vi "ReportPart.vi"(6 "试验项目":T2(ring), 8 "error in":errorcluster, 9 "索引IN":i32, 10 "合格":T1, 11 "report in":refnum<class "NI_report.lvclass">) -> (0 "error out 2":errorcluster caption="error out", 2 "索引OUT":i32, 3 "report out":refnum<class "NI_report.lvclass">)   [LabVIEW 2020]
uses:
  <vilib>/Utility/NIReport.llb/NI_report.lvclass
  OK.ctl
  <vilib>/Utility/NIReport.llb/image depth.ctl
  <vilib>/addons/_office/_exclsub.llb/font.ctl
  Global_Variable/Global.vi
  Global_Variable/A180648.vi
  <vilib>/Utility/NIReport.llb/Append Report Text (str wrap).vi
  <vilib>/addons/_office/word.llb/Word Easy Table (str).vi
  <vilib>/Utility/NIReport.llb/NI_ReportGenerationCore.lvlib
  <vilib>/addons/_office/NI_ReportGenerationToolkit.lvlib
  <vilib>/Utility/NIReport.llb/Word/NI_Word.lvclass
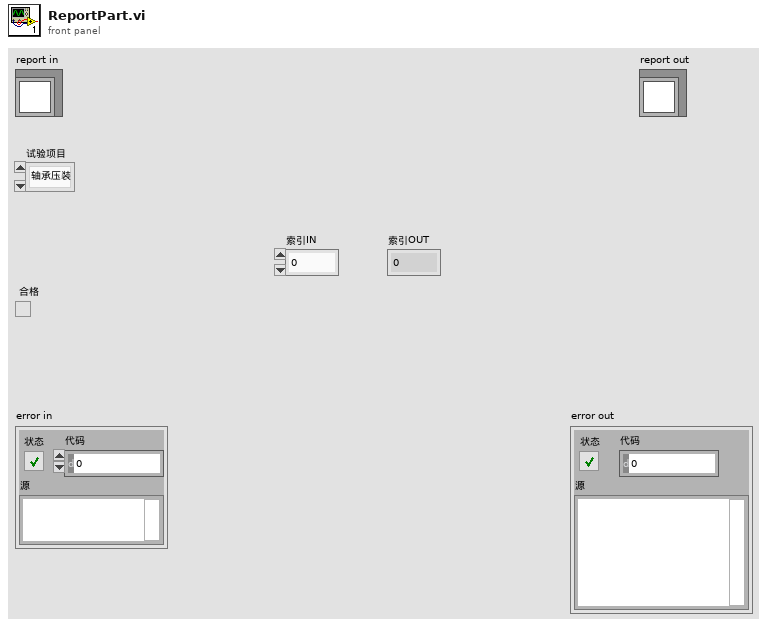
[diagram p1: front panel]
types:
  T1 = typedef "OK.ctl" = bool
  T2 = enum32{"轴承压装", "侧铆", "端铆", "电流特性", "传感器特性", "振动NVH", "磨合"}
  T3 = cluster{"Charset (-1)":i16, "Weight (-1)":i16, "Name":string, "Size":string}
  T4 = typedef "NI_ReportGenerationToolkit.lvlib/font.ctl" = cluster{"font name":string, "font size":dbl, "bold":u16, "italic":u16, "underline":u16, "strike through":u16, "font color":u32}
  T5 = cluster{"Italic":enum16{"Italic Unchanged", "Italic On", "Italic Off"}, "Strike Through":enum16{"Strike Through Unchanged", "Strike Through On", "Strike Through Off"}, "Underline":enum16{"Underline Unchanged", "Underline On", "Underline Off"}, "Bold":enum16{"Bold Unchanged", "Bold On", "Bold Off"}}
  T6 = typedef "NI_ReportGenerationCore.lvlib/image depth.ctl" = u16
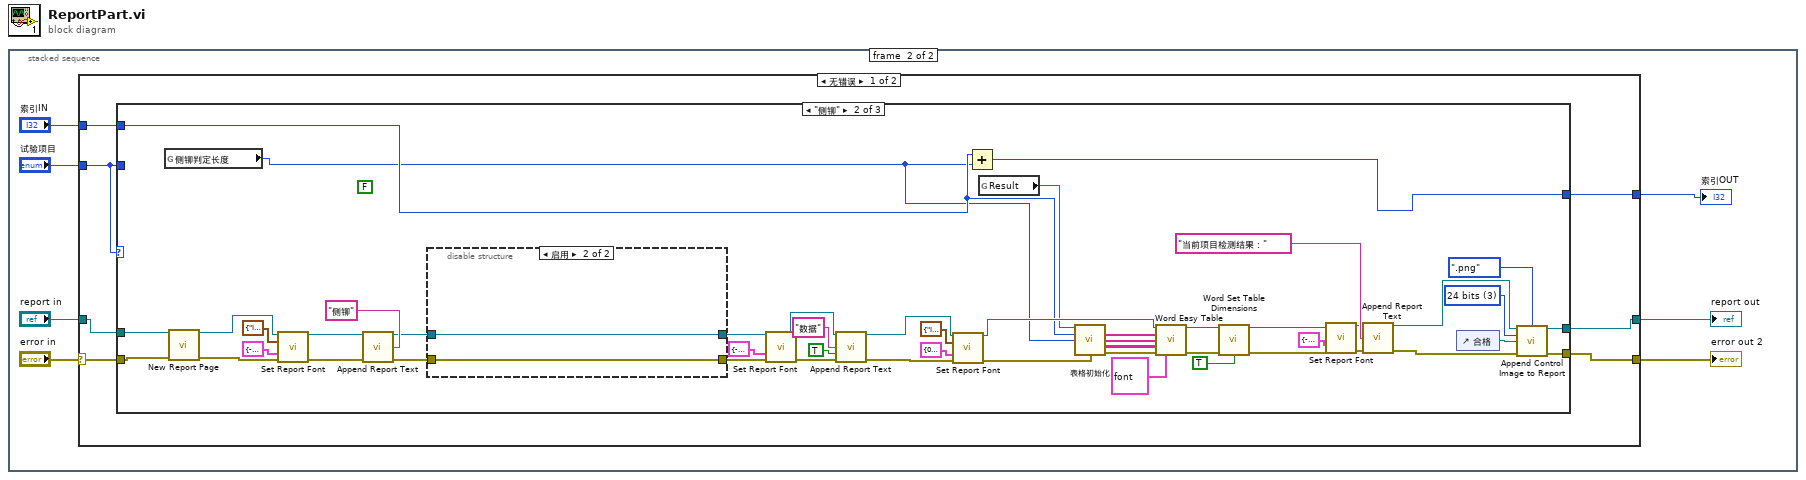
[diagram p0: block diagram]
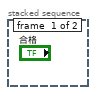
[diagram p2: hidden frame]
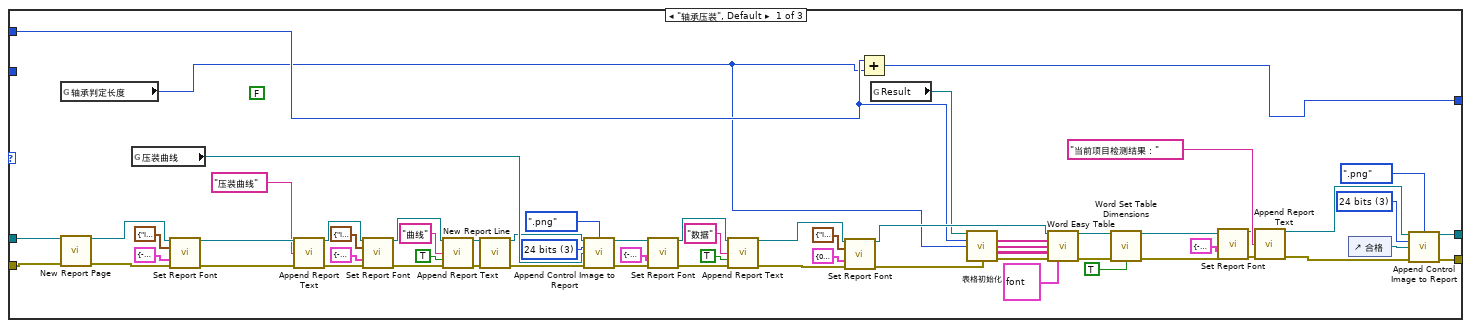
[diagram p3: hidden frame]
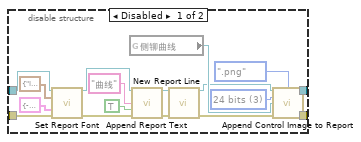
[diagram p4: hidden frame]
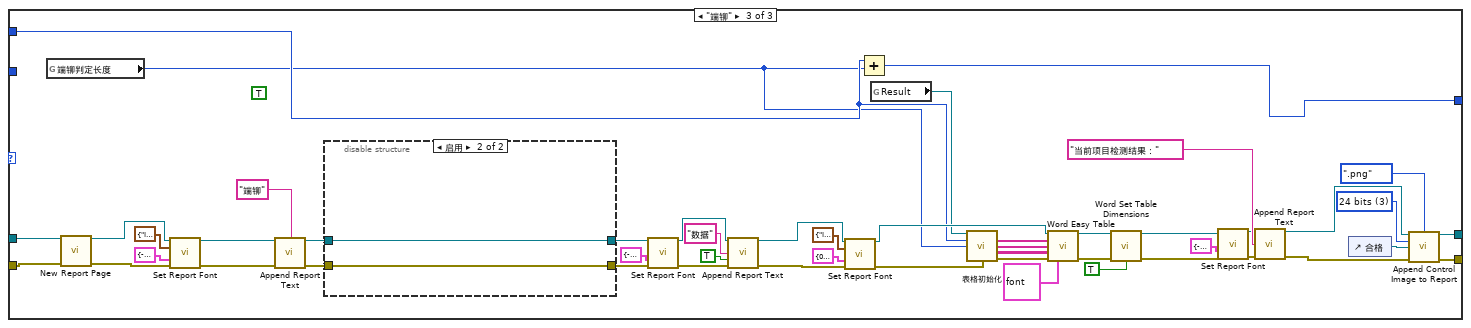
[diagram p5: hidden frame]
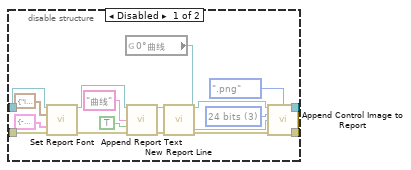
[diagram p6: hidden frame]
diagram:
  n1 = stacked-sequence {
    frame #0 {
    }
    frame #1 {
      n2 = case shown="无错误" "error in" {
        selector: "error in" -> [w14 w215]
        tunnel: [w13 w215] -> w6
        tunnel: "索引IN" -> [w9 w213]
        tunnel: "试验项目" -> [w8 _]
        tunnel: [w10 w213] -> w1
        tunnel: [w12 w214] -> w3
        tunnel: "report in" -> [w11 w214]
        frame No Error {
          n3 = case shown="\"侧铆\"" w8 {
            tunnel: w14 -> [w69 w118 w186]
            tunnel: [w64 w113 w181] -> w13
            tunnel: w8 -> [_ _ _]
            tunnel: [w39 w101 w169] -> w12
            tunnel: w11 -> [w38 w100 w168]
            tunnel: [w36 w98 w166] -> w10
            tunnel: w9 -> [w16 w78 w146]
            frame "轴承压装", Default {
              (unwired) FALSE
              w52 = T6 3 items=["B&W", "4 bits", "8 bits", "24 bits"] ("image depth")
              w62 = T6 3 items=["B&W", "4 bits", "8 bits", "24 bits"] ("image depth")
              n4 = global read "判定参数.vi" "轴承判定长度"() -> (w15:i32)
              n5 = call-dynamic "New Report Page.vi"("report in"=w38, "error in (no error)"=w69) -> ("report out"=w67:refnum<class "NI_report.lvclass">, "error out"=w68:errorcluster)  [unwired: 12 in]
              n6 = global read "A180648.vi" "压装曲线"() -> (w55:refnum<vi>)
              n7 = call-dynamic "Set Report Font.vi"("report in"=w67, "text options"=T5 {"Italic"=enum."Italic Unchanged", "Strike Through"=enum."Strike Through Unchanged", "Underline"=enum."Underline Unchanged", "Bold"=enum."Bold On"}, "font settings"=T3 {"Charset (-1)"=-1, "Weight (-1)"=-1, "Name"="楷体", "Size"="16 "}, "error in (no error)"=w68) -> ("report out"=w76:refnum<class "NI_report.lvclass">, "error out"=w75:errorcluster)  [unwired: 9 in, 1 out]
              n8 = call-poly <vilib>:"Append Report Text.vi"("report in"=w76, "text"="压装曲线", "error in (no error)"=w75) -> ("report out"=w71:refnum<class "NI_report.lvclass">, "error out"=w70:errorcluster)  [unwired: 9 in, 2 out]
              n9 = call-dynamic "Set Report Font.vi"("report in"=w71, "text options"=T5 {"Italic"=enum."Italic Unchanged", "Strike Through"=enum."Strike Through Unchanged", "Underline"=enum."Underline Unchanged", "Bold"=enum."Bold Off"}, "font settings"=T3 {"Charset (-1)"=-1, "Weight (-1)"=-1, "Name"="宋体", "Size"="12"}, "error in (no error)"=w70) -> ("report out"=w46:refnum<class "NI_report.lvclass">, "error out"=w43:errorcluster)  [unwired: 9 in, 1 out]
              n10 = call-poly <vilib>:"Append Report Text.vi"("report in"=w46, "text"="曲线", "append on new line? (F)"=TRUE, "error in (no error)"=w43) -> ("report out"=w45:refnum<class "NI_report.lvclass">, "error out"=w44:errorcluster)  [unwired: 8 in, 2 out]
              n11 = call-dynamic "New Report Line.vi"("report in"=w45, "error in (no error)"=w44) -> ("report out"=w53:refnum<class "NI_report.lvclass">, "error out"=w54:errorcluster)  [unwired: 12 in]
              n12 = call-dynamic "Append Control Image to Report.vi"("report in"=w53, "image file type (.jpg)"=enum16{".jpg", ".png"}.".png", "image depth"=w52, "ctrl reference"=w55, "error in (no error)"=w54) -> ("report out"=w50:refnum<class "NI_report.lvclass">, "error out"=w49:errorcluster)  [unwired: 7 in, 2 out]
              n13 = call-dynamic "Set Report Font.vi"("report in"=w50, "font settings"=T3 {"Charset (-1)"=-1, "Weight (-1)"=-1, "Name"="微软雅黑", "Size"="12 "}, "error in (no error)"=w49) -> ("report out"=w35:refnum<class "NI_report.lvclass">, "error out"=w32:errorcluster)  [unwired: 10 in, 1 out]
              n14 = call-poly <vilib>:"Append Report Text.vi"("report in"=w35, "text"="数据", "append on new line? (F)"=TRUE, "error in (no error)"=w32) -> ("report out"=w18:refnum<class "NI_report.lvclass">, "error out"=w17:errorcluster)  [unwired: 8 in, 2 out]
              n15 = call-dynamic "Set Report Font.vi"("report in"=w18, "text options"=T5 {"Italic"=enum."Italic Unchanged", "Strike Through"=enum."Strike Through Unchanged", "Underline"=enum."Underline Unchanged", "Bold"=enum."Bold Unchanged"}, "font settings"=T3 {"Charset (-1)"=0, "Weight (-1)"=-1, "Name"="微软雅黑", "Size"="12 "}, "error in (no error)"=w17) -> ("report out"=w21:refnum<class "NI_report.lvclass">, "error out"=w20:errorcluster)  [unwired: 9 in, 1 out]
              n16 = Add(x=w16, y=w15) -> (x+y=w36:i32)
              n17 = global read "Global.vi" "Result"() -> (w19:refnum<vi>)
              n18 = call "表格初始化.vi"("表格引用"=w19, "索引"=w16, "长度"=w15, "错误输入（无错误）"=w20) -> ("行首字符串[]"=w23:string[], "列首字符串[]"=w22:string[], "文本数据"=w25:string[][], "错误输出"=w28:errorcluster)  [unwired: 7 in, 1 out]
              n19 = call-poly <vilib>:"Word Easy Table.vi"("report in"=w21, "row headers"=w23, "column headers"=w22, "data"=w25, "error in (no error)"=w28, "font"=T4 {"font name"="宋体", "font size"=12.0, "bold"=2, "italic"=2, "underline"=2, "strike through"=2, "font color"=16777216}) -> ("report out"=w26:refnum<class "NI_report.lvclass">, "error out"=w27:errorcluster)  [unwired: 7 in, 1 out]
              n20 = call <vilib>:"Word Set Table Dimensions.vi"("report in"=w26, "error in (no error)"=w27, "fit to page width? (F)"=TRUE) -> ("report out"=w57:refnum<class "NI_report.lvclass">, "error out"=w56:errorcluster)  [unwired: 11 in]
              n21 = call-dynamic "Set Report Font.vi"("report in"=w57, "font settings"=T3 {"Charset (-1)"=-1, "Weight (-1)"=-1, "Name"="宋体", "Size"="16 "}, "error in (no error)"=w56) -> ("report out"=w60:refnum<class "NI_report.lvclass">, "error out"=w61:errorcluster)  [unwired: 10 in, 1 out]
              n22 = call-poly <vilib>:"Append Report Text.vi"("report in"=w60, "text"="当前项目检测结果：", "error in (no error)"=w61) -> ("report out"=w66:refnum<class "NI_report.lvclass">, "error out"=w65:errorcluster)  [unwired: 9 in, 2 out]
              n23 = control-ref of="合格"() -> (w37:refnum<vi>)
              n24 = call-dynamic "Append Control Image to Report.vi"("report in"=w66, "image file type (.jpg)"=enum16{".jpg", ".png"}.".png", "image depth"=w62, "ctrl reference"=w37, "error in (no error)"=w65) -> ("report out"=w39:refnum<class "NI_report.lvclass">, "error out"=w64:errorcluster)  [unwired: 7 in, 2 out]
            }
            frame "侧铆" {
              (unwired) FALSE
              w111 = T6 3 items=["B&W", "4 bits", "8 bits", "24 bits"] ("image depth")
              n25 = global read "判定参数.vi" "侧铆判定长度"() -> (w77:i32)
              n26 = call-dynamic "New Report Page.vi"("report in"=w100, "error in (no error)"=w118) -> ("report out"=w116:refnum<class "NI_report.lvclass">, "error out"=w117:errorcluster)  [unwired: 12 in]
              n27 = call-dynamic "Set Report Font.vi"("report in"=w116, "text options"=T5 {"Italic"=enum."Italic Unchanged", "Strike Through"=enum."Strike Through Unchanged", "Underline"=enum."Underline Unchanged", "Bold"=enum."Bold On"}, "font settings"=T3 {"Charset (-1)"=-1, "Weight (-1)"=-1, "Name"="楷体", "Size"="16 "}, "error in (no error)"=w117) -> ("report out"=w125:refnum<class "NI_report.lvclass">, "error out"=w124:errorcluster)  [unwired: 9 in, 1 out]
              n28 = call-poly <vilib>:"Append Report Text.vi"("report in"=w125, "text"="侧铆", "error in (no error)"=w124) -> ("report out"=w120:refnum<class "NI_report.lvclass">, "error out"=w119:errorcluster)  [unwired: 9 in, 2 out]
              n29 = disable-structure shown="启用" {
                disable-tunnel: w120 -> [w142 w144]
                disable-tunnel: w119 -> [w141 w143]
                disable-tunnel: [w136 w144] -> w103
                disable-tunnel: [w135 w143] -> w102
                frame Disabled {
                  w137 = T6 3 items=["B&W", "4 bits", "8 bits", "24 bits"] ("image depth")
                  n30 = call-dynamic "Set Report Font.vi"("report in"=w142, "text options"=T5 {"Italic"=enum."Italic Unchanged", "Strike Through"=enum."Strike Through Unchanged", "Underline"=enum."Underline Unchanged", "Bold"=enum."Bold Off"}, "font settings"=T3 {"Charset (-1)"=-1, "Weight (-1)"=-1, "Name"="宋体", "Size"="12"}, "error in (no error)"=w141) -> ("report out"=w132:refnum<class "NI_report.lvclass">, "error out"=w129:errorcluster)  [unwired: 9 in, 1 out]
                  n31 = global read "A180648.vi" "侧铆曲线"() -> (w140:refnum<vi>)
                  n32 = call-poly <vilib>:"Append Report Text.vi"("report in"=w132, "text"="曲线", "append on new line? (F)"=TRUE, "error in (no error)"=w129) -> ("report out"=w131:refnum<class "NI_report.lvclass">, "error out"=w130:errorcluster)  [unwired: 8 in, 2 out]
                  n33 = call-dynamic "New Report Line.vi"("report in"=w131, "error in (no error)"=w130) -> ("report out"=w138:refnum<class "NI_report.lvclass">, "error out"=w139:errorcluster)  [unwired: 12 in]
                  n34 = call-dynamic "Append Control Image to Report.vi"("report in"=w138, "image file type (.jpg)"=enum16{".jpg", ".png"}.".png", "image depth"=w137, "ctrl reference"=w140, "error in (no error)"=w139) -> ("report out"=w136:refnum<class "NI_report.lvclass">, "error out"=w135:errorcluster)  [unwired: 7 in, 2 out]
                }
                frame Enabled {
                }
              }
              n35 = call-dynamic "Set Report Font.vi"("report in"=w103, "font settings"=T3 {"Charset (-1)"=-1, "Weight (-1)"=-1, "Name"="微软雅黑", "Size"="12 "}, "error in (no error)"=w102) -> ("report out"=w97:refnum<class "NI_report.lvclass">, "error out"=w94:errorcluster)  [unwired: 10 in, 1 out]
              n36 = call-poly <vilib>:"Append Report Text.vi"("report in"=w97, "text"="数据", "append on new line? (F)"=TRUE, "error in (no error)"=w94) -> ("report out"=w80:refnum<class "NI_report.lvclass">, "error out"=w79:errorcluster)  [unwired: 8 in, 2 out]
              n37 = call-dynamic "Set Report Font.vi"("report in"=w80, "text options"=T5 {"Italic"=enum."Italic Unchanged", "Strike Through"=enum."Strike Through Unchanged", "Underline"=enum."Underline Unchanged", "Bold"=enum."Bold Unchanged"}, "font settings"=T3 {"Charset (-1)"=0, "Weight (-1)"=-1, "Name"="微软雅黑", "Size"="12 "}, "error in (no error)"=w79) -> ("report out"=w83:refnum<class "NI_report.lvclass">, "error out"=w82:errorcluster)  [unwired: 9 in, 1 out]
              n38 = Add(x=w78, y=w77) -> (x+y=w98:i32)
              n39 = global read "Global.vi" "Result"() -> (w81:refnum<vi>)
              n40 = call "表格初始化.vi"("表格引用"=w81, "索引"=w78, "长度"=w77, "错误输入（无错误）"=w82) -> ("行首字符串[]"=w85:string[], "列首字符串[]"=w84:string[], "文本数据"=w87:string[][], "错误输出"=w90:errorcluster)  [unwired: 7 in, 1 out]
              n41 = call-poly <vilib>:"Word Easy Table.vi"("report in"=w83, "row headers"=w85, "column headers"=w84, "data"=w87, "error in (no error)"=w90, "font"=T4 {"font name"="宋体", "font size"=12.0, "bold"=2, "italic"=2, "underline"=2, "strike through"=2, "font color"=16777216}) -> ("report out"=w88:refnum<class "NI_report.lvclass">, "error out"=w89:errorcluster)  [unwired: 7 in, 1 out]
              n42 = call <vilib>:"Word Set Table Dimensions.vi"("report in"=w88, "error in (no error)"=w89, "fit to page width? (F)"=TRUE) -> ("report out"=w106:refnum<class "NI_report.lvclass">, "error out"=w105:errorcluster)  [unwired: 11 in]
              n43 = call-dynamic "Set Report Font.vi"("report in"=w106, "font settings"=T3 {"Charset (-1)"=-1, "Weight (-1)"=-1, "Name"="宋体", "Size"="16 "}, "error in (no error)"=w105) -> ("report out"=w109:refnum<class "NI_report.lvclass">, "error out"=w110:errorcluster)  [unwired: 10 in, 1 out]
              n44 = call-poly <vilib>:"Append Report Text.vi"("report in"=w109, "text"="当前项目检测结果：", "error in (no error)"=w110) -> ("report out"=w115:refnum<class "NI_report.lvclass">, "error out"=w114:errorcluster)  [unwired: 9 in, 2 out]
              n45 = control-ref of="合格"() -> (w99:refnum<vi>)
              n46 = call-dynamic "Append Control Image to Report.vi"("report in"=w115, "image file type (.jpg)"=enum16{".jpg", ".png"}.".png", "image depth"=w111, "ctrl reference"=w99, "error in (no error)"=w114) -> ("report out"=w101:refnum<class "NI_report.lvclass">, "error out"=w113:errorcluster)  [unwired: 7 in, 2 out]
            }
            frame "端铆" {
              (unwired) TRUE
              w179 = T6 3 items=["B&W", "4 bits", "8 bits", "24 bits"] ("image depth")
              n47 = global read "判定参数.vi" "端铆判定长度"() -> (w145:i32)
              n48 = call-dynamic "New Report Page.vi"("report in"=w168, "error in (no error)"=w186) -> ("report out"=w184:refnum<class "NI_report.lvclass">, "error out"=w185:errorcluster)  [unwired: 12 in]
              n49 = call-dynamic "Set Report Font.vi"("report in"=w184, "text options"=T5 {"Italic"=enum."Italic Unchanged", "Strike Through"=enum."Strike Through Unchanged", "Underline"=enum."Underline Unchanged", "Bold"=enum."Bold On"}, "font settings"=T3 {"Charset (-1)"=-1, "Weight (-1)"=-1, "Name"="楷体", "Size"="16 "}, "error in (no error)"=w185) -> ("report out"=w193:refnum<class "NI_report.lvclass">, "error out"=w192:errorcluster)  [unwired: 9 in, 1 out]
              n50 = call-poly <vilib>:"Append Report Text.vi"("report in"=w193, "text"="端铆", "error in (no error)"=w192) -> ("report out"=w188:refnum<class "NI_report.lvclass">, "error out"=w187:errorcluster)  [unwired: 9 in, 2 out]
              n51 = disable-structure shown="启用" {
                disable-tunnel: w188 -> [w210 w212]
                disable-tunnel: w187 -> [w209 w211]
                disable-tunnel: [w204 w212] -> w171
                disable-tunnel: [w203 w211] -> w170
                frame Disabled {
                  w205 = T6 3 items=["B&W", "4 bits", "8 bits", "24 bits"] ("image depth")
                  n52 = call-dynamic "Set Report Font.vi"("report in"=w210, "text options"=T5 {"Italic"=enum."Italic Unchanged", "Strike Through"=enum."Strike Through Unchanged", "Underline"=enum."Underline Unchanged", "Bold"=enum."Bold Off"}, "font settings"=T3 {"Charset (-1)"=-1, "Weight (-1)"=-1, "Name"="宋体", "Size"="12"}, "error in (no error)"=w209) -> ("report out"=w200:refnum<class "NI_report.lvclass">, "error out"=w197:errorcluster)  [unwired: 9 in, 1 out]
                  n53 = global read "A180648.vi" "0°曲线"() -> (w208:refnum<vi>)
                  n54 = call-poly <vilib>:"Append Report Text.vi"("report in"=w200, "text"="曲线", "append on new line? (F)"=TRUE, "error in (no error)"=w197) -> ("report out"=w199:refnum<class "NI_report.lvclass">, "error out"=w198:errorcluster)  [unwired: 8 in, 2 out]
                  n55 = call-dynamic "New Report Line.vi"("report in"=w199, "error in (no error)"=w198) -> ("report out"=w206:refnum<class "NI_report.lvclass">, "error out"=w207:errorcluster)  [unwired: 12 in]
                  n56 = call-dynamic "Append Control Image to Report.vi"("report in"=w206, "image file type (.jpg)"=enum16{".jpg", ".png"}.".png", "image depth"=w205, "ctrl reference"=w208, "error in (no error)"=w207) -> ("report out"=w204:refnum<class "NI_report.lvclass">, "error out"=w203:errorcluster)  [unwired: 7 in, 2 out]
                }
                frame Enabled {
                }
              }
              n57 = call-dynamic "Set Report Font.vi"("report in"=w171, "font settings"=T3 {"Charset (-1)"=-1, "Weight (-1)"=-1, "Name"="微软雅黑", "Size"="12 "}, "error in (no error)"=w170) -> ("report out"=w165:refnum<class "NI_report.lvclass">, "error out"=w162:errorcluster)  [unwired: 10 in, 1 out]
              n58 = call-poly <vilib>:"Append Report Text.vi"("report in"=w165, "text"="数据", "append on new line? (F)"=TRUE, "error in (no error)"=w162) -> ("report out"=w148:refnum<class "NI_report.lvclass">, "error out"=w147:errorcluster)  [unwired: 8 in, 2 out]
              n59 = call-dynamic "Set Report Font.vi"("report in"=w148, "text options"=T5 {"Italic"=enum."Italic Unchanged", "Strike Through"=enum."Strike Through Unchanged", "Underline"=enum."Underline Unchanged", "Bold"=enum."Bold Unchanged"}, "font settings"=T3 {"Charset (-1)"=0, "Weight (-1)"=-1, "Name"="微软雅黑", "Size"="12 "}, "error in (no error)"=w147) -> ("report out"=w151:refnum<class "NI_report.lvclass">, "error out"=w150:errorcluster)  [unwired: 9 in, 1 out]
              n60 = Add(x=w146, y=w145) -> (x+y=w166:i32)
              n61 = global read "Global.vi" "Result"() -> (w149:refnum<vi>)
              n62 = call "表格初始化.vi"("表格引用"=w149, "索引"=w146, "长度"=w145, "错误输入（无错误）"=w150) -> ("行首字符串[]"=w153:string[], "列首字符串[]"=w152:string[], "文本数据"=w155:string[][], "错误输出"=w158:errorcluster)  [unwired: 7 in, 1 out]
              n63 = call-poly <vilib>:"Word Easy Table.vi"("report in"=w151, "row headers"=w153, "column headers"=w152, "data"=w155, "error in (no error)"=w158, "font"=T4 {"font name"="宋体", "font size"=12.0, "bold"=2, "italic"=2, "underline"=2, "strike through"=2, "font color"=16777216}) -> ("report out"=w156:refnum<class "NI_report.lvclass">, "error out"=w157:errorcluster)  [unwired: 7 in, 1 out]
              n64 = call <vilib>:"Word Set Table Dimensions.vi"("report in"=w156, "error in (no error)"=w157, "fit to page width? (F)"=TRUE) -> ("report out"=w174:refnum<class "NI_report.lvclass">, "error out"=w173:errorcluster)  [unwired: 11 in]
              n65 = call-dynamic "Set Report Font.vi"("report in"=w174, "font settings"=T3 {"Charset (-1)"=-1, "Weight (-1)"=-1, "Name"="宋体", "Size"="16 "}, "error in (no error)"=w173) -> ("report out"=w177:refnum<class "NI_report.lvclass">, "error out"=w178:errorcluster)  [unwired: 10 in, 1 out]
              n66 = call-poly <vilib>:"Append Report Text.vi"("report in"=w177, "text"="当前项目检测结果：", "error in (no error)"=w178) -> ("report out"=w183:refnum<class "NI_report.lvclass">, "error out"=w182:errorcluster)  [unwired: 9 in, 2 out]
              n67 = control-ref of="合格"() -> (w167:refnum<vi>)
              n68 = call-dynamic "Append Control Image to Report.vi"("report in"=w183, "image file type (.jpg)"=enum16{".jpg", ".png"}.".png", "image depth"=w179, "ctrl reference"=w167, "error in (no error)"=w182) -> ("report out"=w169:refnum<class "NI_report.lvclass">, "error out"=w181:errorcluster)  [unwired: 7 in, 2 out]
            }
          }
        }
        frame Error {
        }
      }
      "error out 2" <- w6
      "索引OUT" <- w1
      "report out" <- w3
    }
  }
